vi "Graph ERD Read List.vi"(0 "GEA2 Reference In":refnum<k24>, 5 "GEA Inputs":T10={"Source"=240, "Destination"=35} {"Destination" format="%.0x"; "Source" format="%.0x"}, 7 "ERD_Data_Bundled_In":T1, 9 "ERD Graph Cntrl":T11={"ERD 3"={"ERD #"=0, "Data Type"=enum."uint16_t", "Scaler"=1}, "ERD 2"={"ERD #"=0, "Data Type"=enum."uint16_t", "Scaler"=1}, "ERD 1"={"ERD #"=0, "Data Type"=enum."uint16_t", "Scaler"=1}} {"ERD 1"."Scaler" min=1; "ERD 1"."ERD #" format="%.0x"; "ERD 2"."Scaler" min=1; "ERD 2"."ERD #" format="%.0x"; "ERD 3"."Scaler" min=1; "ERD 3"."ERD #" format="%.0x"}, 11 "Error In":errorcluster) -> (4 "GEA2 Reference Out":refnum<k24>, 6 "ERD Graph  Ind":T9, 8 "ERD_Data_Bundled_Out":T1, 15 "Error Out":errorcluster)   [LabVIEW 2016]
uses:
  type defs/ERD_Graph_All.ctl
  type defs/ERD_Graph.ctl
  Common/LabVIEW GEA2 Toolkit/LabVIEW_GEA2_Toolkit.lvlibp/type defs/Data Type.ctl
  Common/LabVIEW GEA2 Toolkit/LabVIEW_GEA2_Toolkit.lvlibp/type defs/Source_Destination.ctl
  type defs/ERD_Data_Bundled.ctl
  type defs/ATC_Data.ctl
  type defs/Redundant.ctl
  type defs/Version.ctl
  type defs/Algorithms.ctl
  type defs/ERD_Always_Show.ctl
  type defs/Fault_Table_Info.ctl
  type defs/Cycle_Diag.ctl
  C:/Automation/DLLs/PC Dot Net/GeaCommunication.dll
  Common/LabVIEW GEA2 Toolkit/LabVIEW_GEA2_Toolkit.lvlibp/type defs/ERD Read Data In.ctl
  Common/LabVIEW GEA2 Toolkit/LabVIEW_GEA2_Toolkit.lvlibp
panel:
  # "Wet Load Size"
  # "Dry Load Size"
  # "OOB"
  # "Software Version"
  # "UI"
  # "MC"
  # "INV"
  # "PERSONALITY"
  # "Wet Load Size"
  # "Dry Load Size"
  # "OOB"
  # "Software Version"
  # "UI"
  # "MC"
  # "INV"
  # "PERSONALITY"
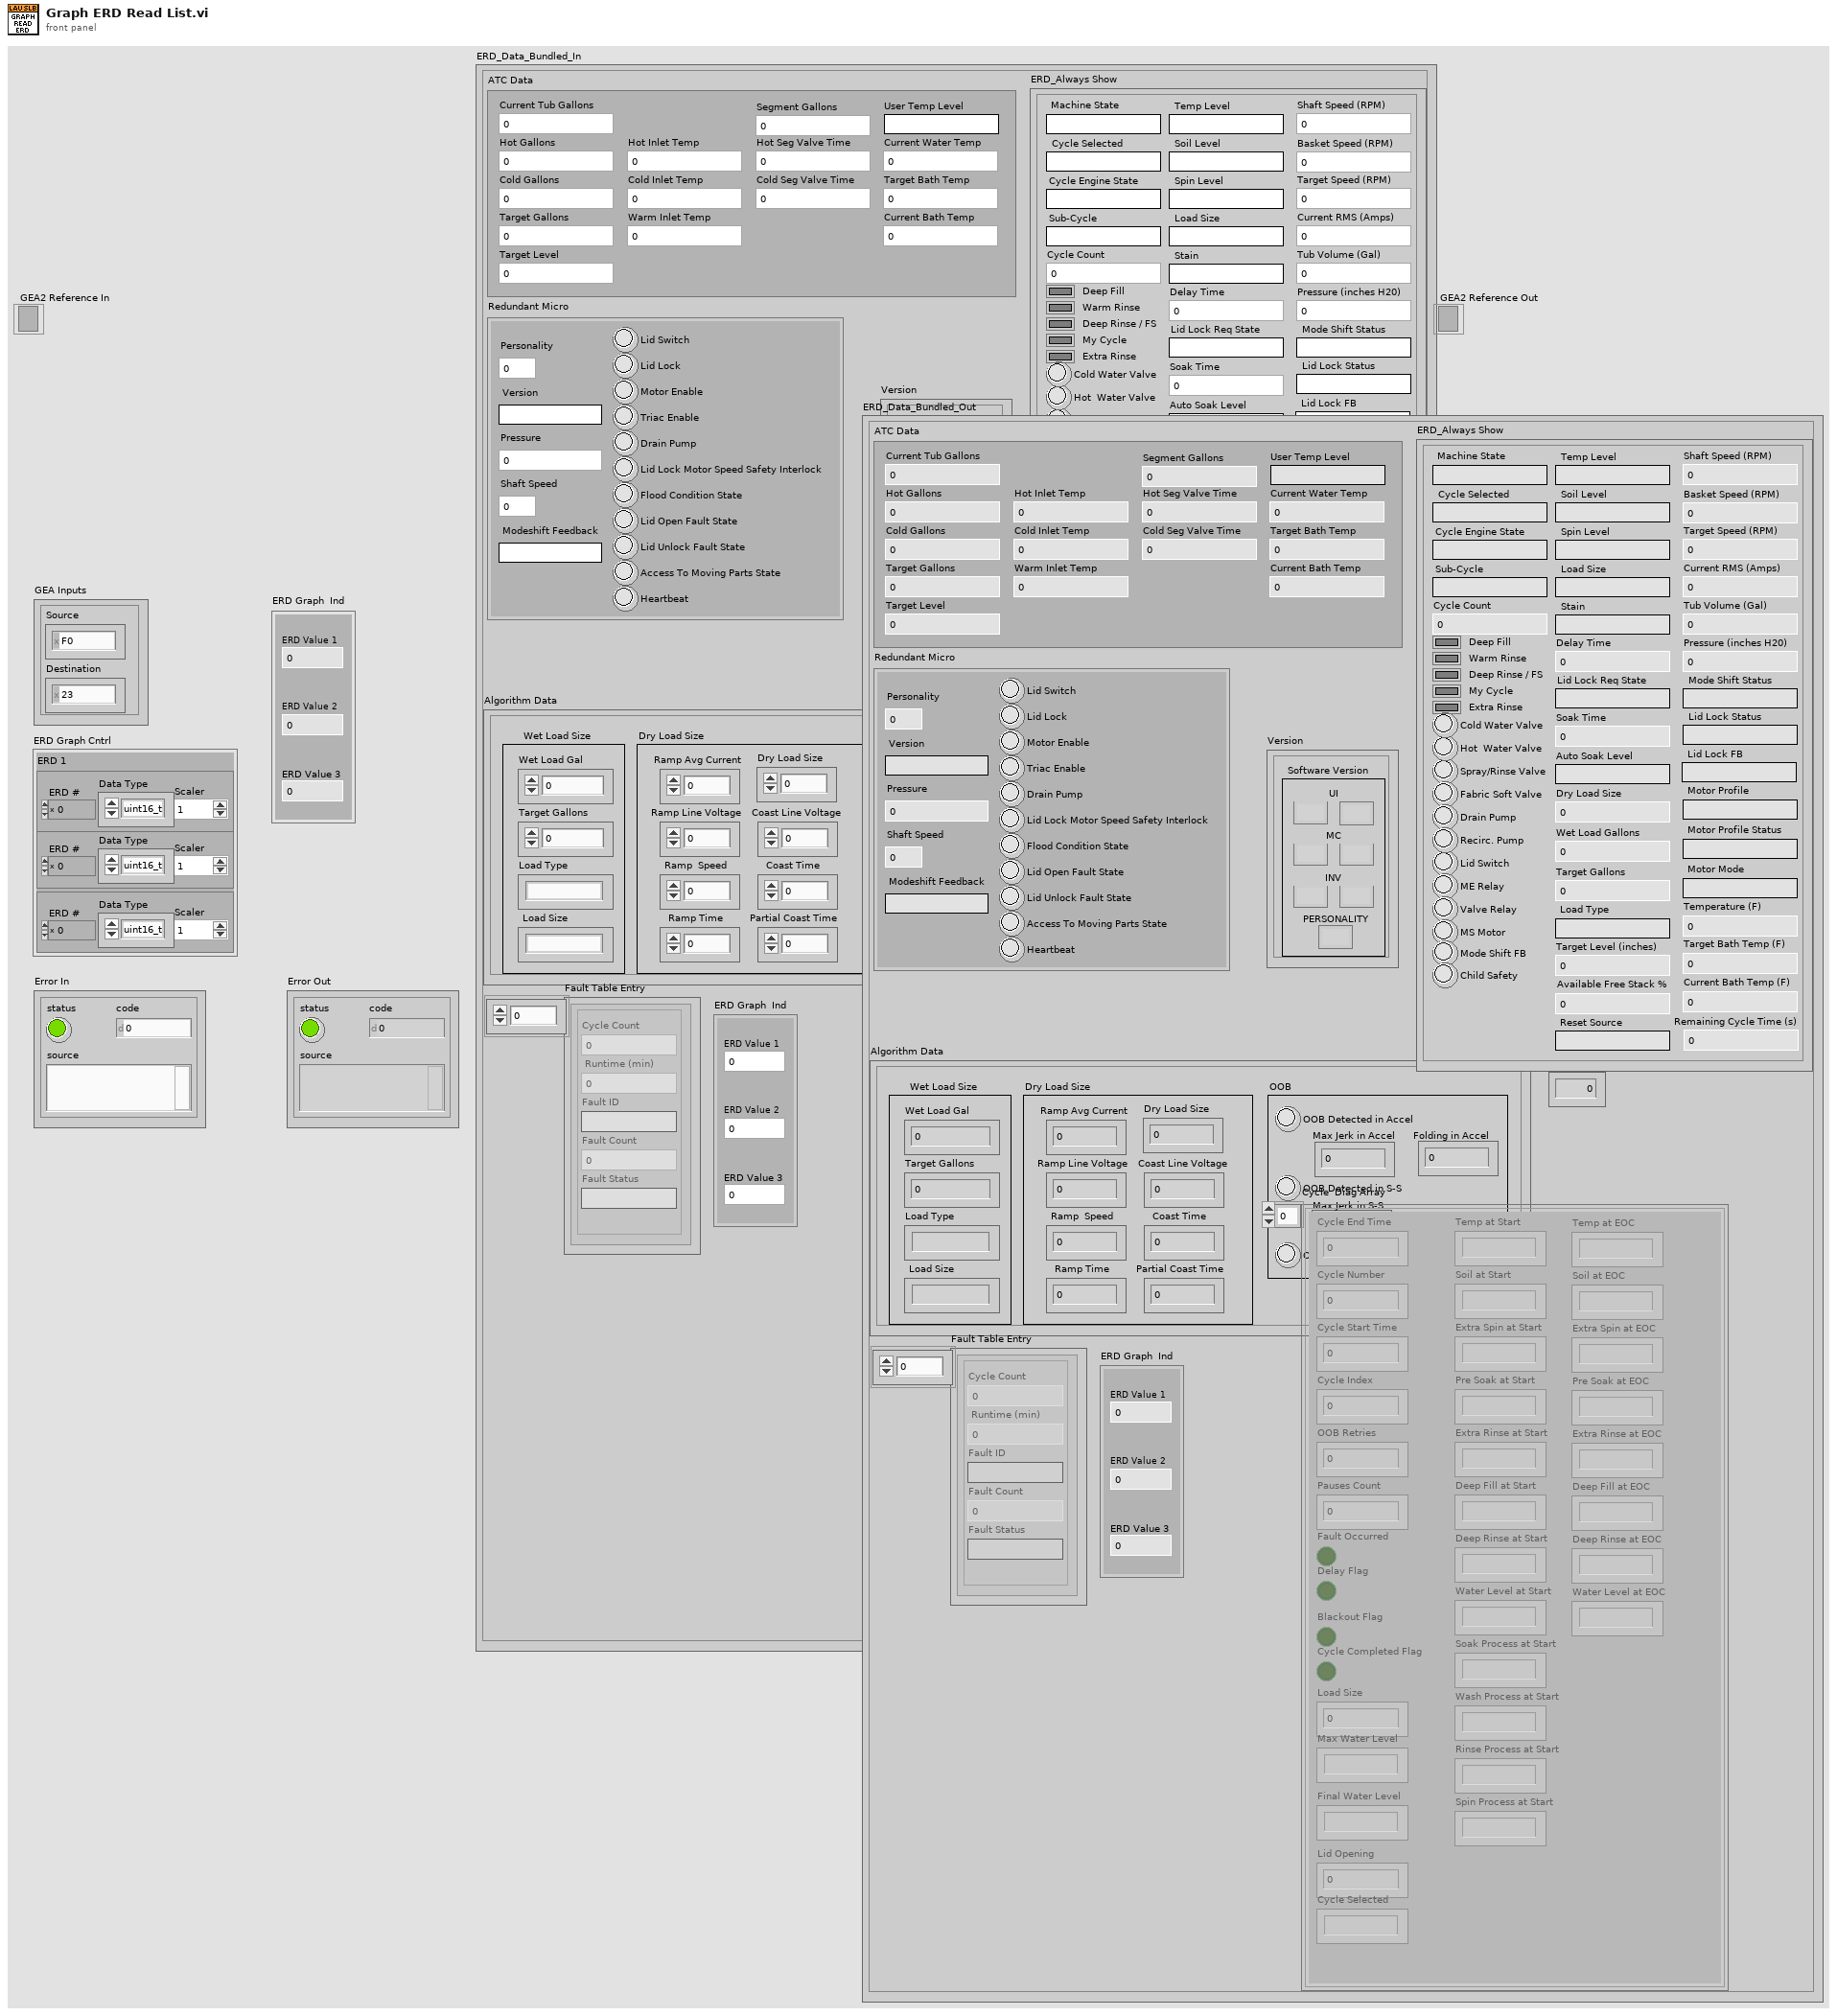
[diagram p1: front panel]
types:
  T1 = typedef "ERD_Data_Bundled.ctl" = cluster{"ATC Data":T2, "Redundant Micro":T3, "Version":T4, "Algorithm Data":T5, "ERD_Always Show":T6, "ERD Graph  Ind":cluster{"ERD Value 1":dbl, "ERD Value 2":dbl, "ERD Value 3":dbl}, "Personality Set":u8, "Fault Table Entry":T7[], "Cycle  Diag Array":T8[]}
  T2 = typedef "ATC_Data.ctl" = cluster{"Current Tub Gallons":dbl, "Hot Gallons":dbl, "Cold Gallons":dbl, "Target Gallons":dbl, "Current Water Temp":dbl, "Target Level":u32, "Target Bath Temp":dbl, "Current Bath Temp ":dbl, "Cold Inlet Temp":dbl, "Hot Inlet Temp":dbl, "Warm Inlet Temp":dbl, "Hot Seg Valve Time":u16, "Cold Seg Valve Time ":u16, "User Temp Level":string, "Segment Gallons":dbl}
  T3 = typedef "Redundant.ctl" = cluster{"Version":string, "Personality":u8, "Pressure ":dbl, "Shaft Speed":u16, "Modeshift Feedback":string, "Lid Switch":bool, "Lid Lock":bool, "Triac Enable":bool, "Drain Pump":bool, "Lid Lock Motor Speed Safety Interlock":bool, "Flood Condition State":bool, "Lid Open Fault State":bool, "Access To Moving Parts State":bool, "Heartbeat":bool, "Motor Enable":bool, "Lid Unlock Fault State":bool}
  T4 = typedef "Version.ctl" = cluster{"UI Major":string, "UI Minor":string, "MC Minor":string, "MC Major":string, "Inverter Minor":string, "Inverter Major":string, "Personality":string}
  T5 = typedef "Algorithms.ctl" = cluster{"Wet Load Gal":dbl, "Target Gallons":dbl, "Load Type":string, "Load Size":string, "Coast Time":u16, "Ramp Time":u16, "Ramp  Speed":u16, "Ramp Avg Current":dbl, "OOB Redist Req":bool, "OOB Detected in S-S":bool, "Folding in Accel":i32, "Max Jerk in Accel":i32, "Max Jerk in S-S":i32, "OOB Detected in Accel":bool, "Partial Coast Time":u16, "Dry Load Size":dbl, "Ramp Line Voltage ":dbl, "Coast Line Voltage":dbl}
  T6 = typedef "ERD_Always_Show.ctl" = cluster{"Basket Speed (RPM)":u16, "Machine State":string, "Tub Volume (Gal)":dbl, "Pressure (inches H20)":dbl, "Lid Switch ":bool, "Current RMS (Amps)":dbl, "Cycle Selected":string, "Lid Lock Status":string, "Mode Shift Status":string, "Spray/Rinse Valve":bool, "Fabric Soft Valve":bool, "Drain Pump":bool, "Recirc. Pump":bool, "Cycle Engine State":string, "Hot  Water Valve":bool, "Cold Water Valve":bool, "Motor Profile":string, "Motor Profile Status":string, "Motor Mode":string, "ME Relay":bool, "Cycle Count":u32, "Deep Rinse / FS":bool, "My Cycle":bool, "Soil Level":string, "Spin Level":string, "Stain":string, "Temp Level":string, "Load Size":string, "Delay Time":u16, "Soak Time":u16, "Deep Fill":bool, "Warm Rinse":bool, "Auto Soak Level":string, "Extra Rinse":bool, "Wet Load Gallons":dbl, "Target Gallons":dbl, "Sub-Cycle":string, "Load Type":string, "Target Level (inches)":u32, "Valve Relay":bool, "Dry Load Size":dbl, "Shaft Speed (RPM) ":u16, "MS Motor":bool, "Mode Shift FB":bool, "Target Bath Temp (F)":dbl, "Temperature (F)":dbl, "Current Bath Temp (F)":dbl, "Lid Lock FB":string, "Lid Lock Req State":string, "Remaining Cycle Time (s)":u32, "Available Free Stack %":u8, "Child Safety":bool, "Target Speed (RPM)":u16, "Reset Source":string}
  T7 = typedef "Fault_Table_Info.ctl" = cluster{"Cycle Count":u32, " Runtime (min) ":u32, "Fault Status":string, "Fault ID":string, "Fault Count":u16}
  T8 = typedef "Cycle_Diag.ctl" = cluster{"Cycle End Time":u32, "Cycle Number":u32, "Cycle Start Time":u32, "Cycle Index":u8, "OOB Retries":u8, "Temp at Start":string, "Soil at Start":string, "Extra Spin at Start":string, "Pre Soak at Start":string, "Extra Rinse at Start":string, "Deep Fill at Start":string, "Deep Rinse at Start":string, "Water Level at Start":string, "Soak Process at Start":string, "Wash Process at Start":string, "Rinse Process at Start":string, "Spin Process at Start":string, "Pauses Count":u8, "Fault Occurred":bool, "Delay Flag":bool, "Blackout Flag":bool, "Cycle Completed Flag":bool, "Temp at EOC":string, "Soil at EOC":string, "Extra Spin at EOC":string, "Pre Soak at EOC":string, "Extra Rinse at EOC":string, "Deep Fill at EOC":string, "Deep Rinse at EOC":string, "Water Level at EOC":string, "Load Size":u8, "Max Water Level":string, "Final Water Level":string, "Lid Opening":u8, "Cycle Selected":string}
  T9 = cluster{"ERD Value 1":dbl, "ERD Value 2":dbl, "ERD Value 3":dbl}
  T10 = typedef "LabVIEW_GEA2_Toolkit.lvlibp/Source_Destination.ctl" = cluster{"Source":u8, "Destination":u8}
  T11 = typedef "ERD_Graph_All.ctl" = cluster{"ERD 3":T12, "ERD 2":T12, "ERD 1":T12}
  T12 = typedef "ERD_Graph.ctl" = cluster{"ERD #":u16, "Data Type":T13, "Scaler":u32}
  T13 = typedef "LabVIEW_GEA2_Toolkit.lvlibp/Data Type.ctl" = enum16{"string", "boolean", "uint8_t", "uint16_t", "uint32_t", "uint64_t", "int8_t", "int16_t", "int32_t", "int64_t"}
  T14 = typedef "LabVIEW_GEA2_Toolkit.lvlibp/ERD Read Data In.ctl" = cluster{"ERD Number":u16, "Data Type":T13}
  T15 = typedef "LabVIEW_GEA2_Toolkit.lvlibp/ERD Read Data Out.ctl" = cluster{"ERD Number":u16, "Data":string}
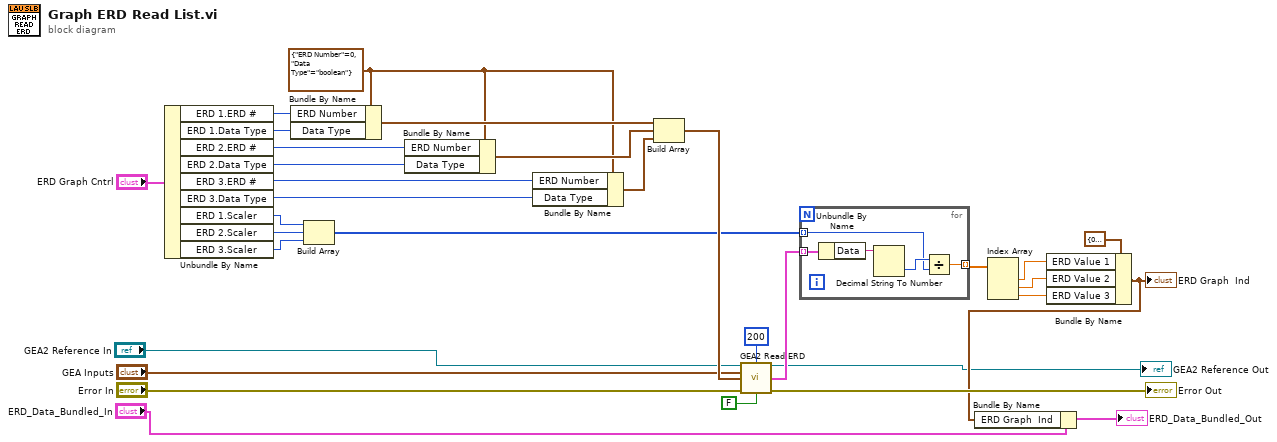
[diagram p0: block diagram]
diagram:
  w28 = T14 {"ERD Number"=0, "Data Type"=enum."boolean"} ("ERD Read Data In 2")
  n1 = Unbundle By Name("ERD Graph Cntrl") -> ("ERD 1.ERD #"=w22:u16, "ERD 1.Data Type"=w23:T13, "ERD 2.ERD #"=w24:u16, "ERD 2.Data Type"=w25:T13, "ERD 3.ERD #"=w26:u16, "ERD 3.Data Type"=w27:T13, "ERD 1.Scaler"=w17:u32, "ERD 2.Scaler"=w16:u32, "ERD 3.Scaler"=w15:u32)
  n2 = Bundle By Name(cluster=w28, "ERD Number"=w22, "Data Type"=w23) -> (w29:T14)
  n3 = Build Array(w17, w16, w15) -> (w14:u32[])
  n4 = Bundle By Name(cluster=w28, "ERD Number"=w24, "Data Type"=w25) -> (w30:T14)
  n5 = Bundle By Name(cluster=w28, "ERD Number"=w26, "Data Type"=w27) -> (w31:T14)
  n6 = Build Array(w29, w30, w31) -> (w21:T14[])
  n7 = call "GEA2 Read ERD.vi"("GEA2 Reference In"="GEA2 Reference In", "Read Timeout (ms)"=u32 200, "GEA Inputs"="GEA Inputs", "Read ERD List"=w21, "Error In"="Error In", "Verify ERD Response?"=FALSE) -> ("GEA2 Reference Out"=→"GEA2 Reference Out":refnum<k24>, "ERD Data Out"=w13:T15[], "Error Out"=→"Error Out":errorcluster)  [unwired: 6 in, 1 out]
  n8 = for {
    tunnel: w14 -> [w34] mode=indexing
    tunnel: w13 -> [w37] mode=indexing
    tunnel: [w33] -> w12 mode=indexing
    n9 = Unbundle By Name(w37) -> ("Data"=w36:string)
    n10 = Decimal String To Number(string=w36) -> (number=w35:i32)  [unwired: 2 in, 1 out]
    n11 = Divide(x=w35, y=w34) -> (x/y=w33:dbl)
  }
  n12 = Index Array(array=w12) -> (element #1=w10:dbl, element #2=w9:dbl, element #3=w8:dbl)  [unwired: 3 in]
  n13 = Bundle By Name(cluster=T9 {"ERD Value 1"=0.0, "ERD Value 2"=0.0, "ERD Value 3"=0.0} ("ERD Graph  Ind"), "ERD Value 1"=w10, "ERD Value 2"=w9, "ERD Value 3"=w8) -> (w4:T9)
  "ERD Graph  Ind" <- w4
  n14 = Bundle By Name(cluster="ERD_Data_Bundled_In", "ERD Graph  Ind"=w4) -> (→"ERD_Data_Bundled_Out":T1)
